vi "Read Mediated Asynchronous Actor.vi"(11 "Last Ack in":refnum<class "Last Ack.lvclass">) -> (2 "Stream Mediator.lvlib:Mediated Asynchronous Actor.lvclass":refnum<class "Mediated Asynchronous Actor.lvclass">, 3 "Last Ack out":refnum<class "Last Ack.lvclass">)   [LabVIEW 2016, in "Stream Mediator.lvlib" / "Last Ack.lvclass"]
uses:
  <userlib>/Composed Systems/Stream/Mediator/Classes/Message Command Last Ack/Last Ack.lvclass
  <userlib>/Composed Systems/Stream/Mediator/Classes/Mediated Asynchronous Actor/Mediated Asynchronous Actor.lvclass
  <userlib>/Composed Systems/Stream/Mediator/Classes/Message Command Last Ack/Last Ack.lvclass/Last Ack.ctl
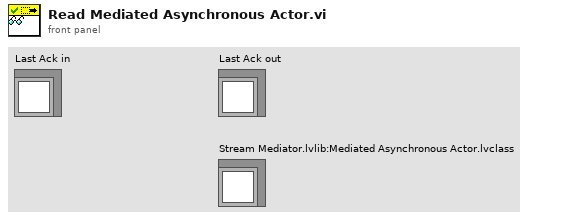
[diagram p1: front panel]
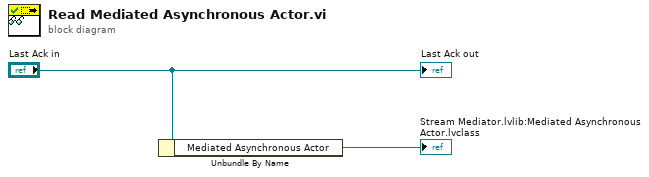
[diagram p0: block diagram]
diagram:
  n1 = Unbundle By Name("Last Ack in") -> ("Mediated Asynchronous Actor"=→"Stream Mediator.lvlib:Mediated Asynchronous Actor.lvclass":refnum<class "Mediated Asynchronous Actor.lvclass">)
  "Last Ack out" <- "Last Ack in"
